vi "未命名 3.vi"() -> ()   [LabVIEW 2017]
panel:
  out "XY图":cluster{dbl[], dbl[]}(graph)
  out "大小 2":i32
  out "大小":i32
  in  "channel group":cluster{"base channel":dbl, "B":dbl}[](array[cluster])=[{"base channel"=10.0, "B"=12.0}, {"base channel"=6.0, "B"=8.0}, {"base channel"=20.0, "B"=22.0}, {"base channel"=24.0, "B"=26.0}, {"base channel"=2.0, "B"=4.0}, {"base channel"=28.0, "B"=30.0}, {"base channel"=16.0, "B"=18.0}, {"base channel"=36.0, "B"=44.0}, {"base channel"=40.0, "B"=42.0}, {"base channel"=32.0, "B"=34.0}]
  in  "TOA":dbl[](graph)=[0.0, 1753.3041851125522, 2130.801088687568, 1436.9138470041964, 2019.919565561429, 1761.4644541054256, 1438.032367974313, 1674.2988778684578, 1531.831940814557, 2230.4923468815937, 5245.493832010657]
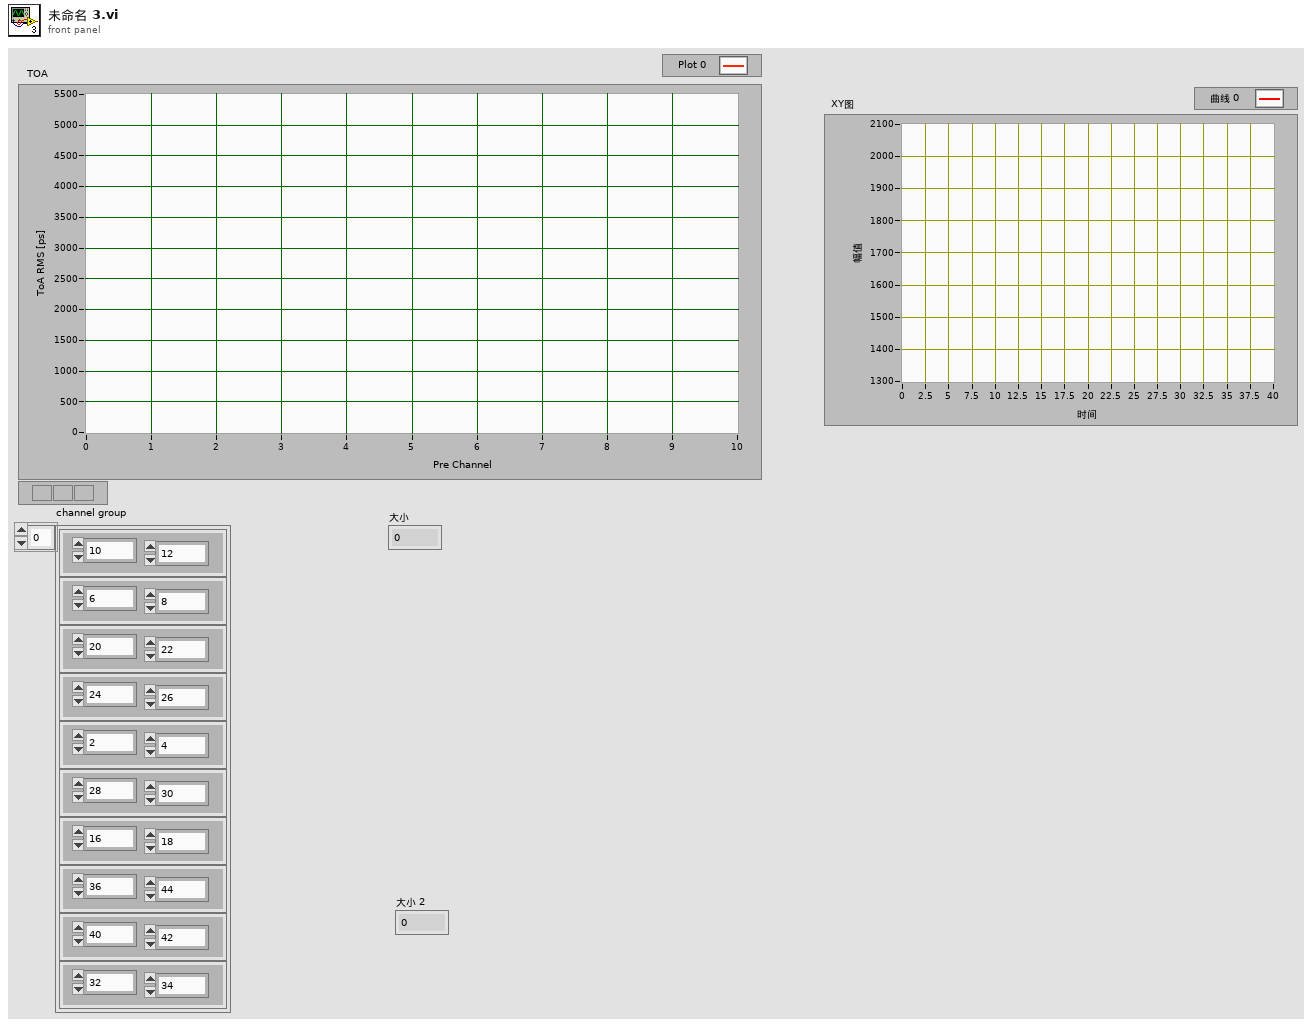
[diagram p1: front panel]
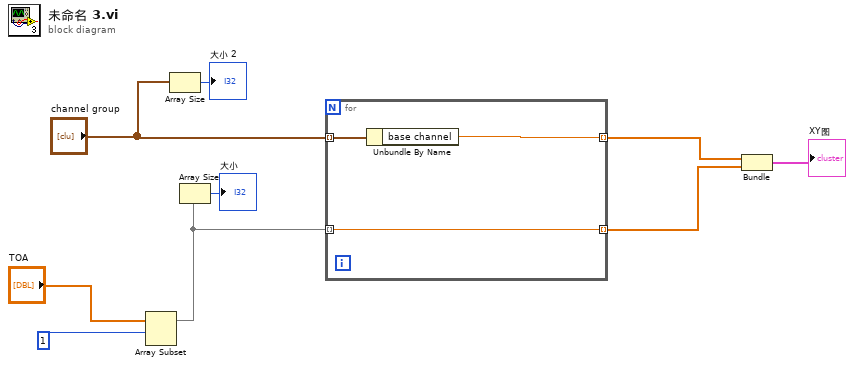
[diagram p0: block diagram]
diagram:
  n1 = Array Subset(array="TOA", index=1 ("索引")) -> (w4:dbl[])  [unwired: 1 in]
  n2 = Array Size(array="channel group") -> (size(s)=→"大小 2":i32)
  n3 = Array Size(array=w4) -> (size(s)=→"大小":i32)
  n4 = for {
    tunnel: "channel group" -> [w11] mode=indexing
    tunnel: w4 -> [w12] mode=indexing
    tunnel: [w12] -> w2 mode=indexing
    tunnel: [w10] -> w3 mode=indexing
    n5 = Unbundle By Name(w11) -> ("base channel"=w10:dbl)
  }
  n6 = Bundle(w3, w2) -> (→"XY图":cluster{dbl[], dbl[]})  [unwired: 1 in]
